vi "GalvosStop.vi"(8 "error in (no error)":errorcluster, 11 "Microscope in":refnum<class "Microscope.lvclass">) -> (0 "error out":errorcluster, 3 "Microscope out":refnum<class "Microscope.lvclass">)   [LabVIEW 2012, in "Microscope.lvclass"]
uses:
  classes/Microscope.lvclass
  classes/Microscope.lvclass/Microscope.ctl
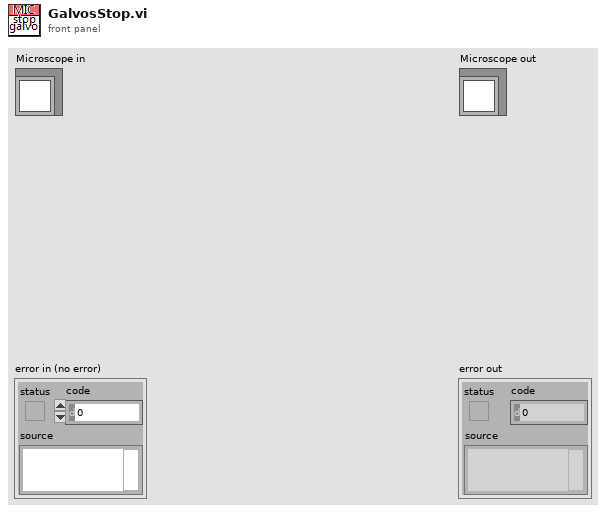
[diagram p1: front panel]
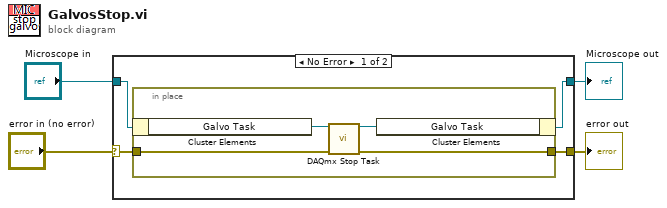
[diagram p0: block diagram]
diagram:
  n1 = case shown="No Error" "error in (no error)" {
    selector: "error in (no error)" -> [w7 w14]
    tunnel: [w6 w14] -> w3
    tunnel: [w5 w13] -> w1
    tunnel: "Microscope in" -> [w8 w13]
    frame No Error {
      n2 = in-place {
        in-place-border: w7 -> [w10]
        in-place-border: [w9] -> w6
        n3 = in-place-cluster #1(w8) -> ("Galvo Task"=w12:refnum<k21>)
        n4 = call <vilib>:"DAQmx Stop Task.vi"("task/channels in"=w12, "error in"=w10) -> ("task out"=w11:refnum<k21>, "error out"=w9:errorcluster)  [unwired: 12 in]
        n5 = in-place-cluster #1("Galvo Task"=w11) -> (w5:refnum<class "Microscope.lvclass">)
      }
    }
    frame Error {
    }
  }
  "error out" <- w3
  "Microscope out" <- w1
